vi "Query Molbloc Range.vi"(8 "error in (no error)":errorcluster, 11 "VISA resource name":refnum<visa-resource-name>) -> (0 "error out":errorcluster, 2 "Molbloc Range":dbl, 3 "VISA resource name out":refnum<visa-resource-name>)   [LabVIEW 2023, in "Fluke Molbox 1 Plus.lvlib"]
doc: "Queries the range designation of the active molbloc. The range designation of the active molbloc is returned in the flow units used to define the range. Note that the effective molbloc range is dependent on the gas being flowed and the molbloc pressure dependent calibration type."
uses:
  Fluke Molbox 1 Plus.lvlib
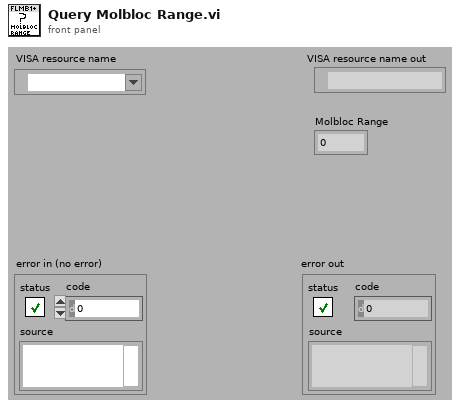
[diagram p1: front panel]
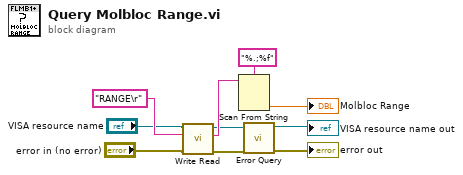
[diagram p0: block diagram]
diagram:
  n1 = call "Write Read.vi"("error in (no error)"="error in (no error)", "Write String"="RANGE\r" ("write buffer"), "VISA resource name"="VISA resource name") -> ("error out"=w3:errorcluster, "Read Response"=w5:string, "VISA resource name out"=w4:refnum<visa-resource-name>)  [unwired: 6 in]
  n2 = Scan From String(format string="%.;%f", input string=w5) -> (output 1=→"Molbloc Range":dbl)  [unwired: 3 in, 3 out]
  n3 = call "Error Query.vi"("error in (no error)"=w3, "VISA resource name"=w4) -> ("error out"=→"error out":errorcluster, "VISA resource name out"=→"VISA resource name out":refnum<visa-resource-name>)  [unwired: 6 in, 2 out]
